vi "Is Enabled.vi"(10 "Plugin in":refnum<class "Plugin.lvclass">) -> (1 "Enabled":bool, 2 "Plugin out":refnum<class "Plugin.lvclass">)   [LabVIEW 2015, in "Plugin.lvclass"]
uses:
  Plugin.lvclass
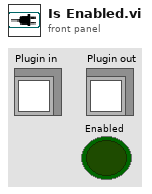
[diagram p1: front panel]
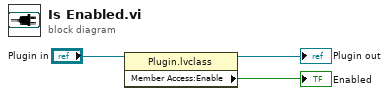
[diagram p0: block diagram]
diagram:
  n1 = property class="Plugin.lvclass"(reference="Plugin in") -> (reference out=→"Plugin out":refnum<class "Plugin.lvclass">, "Member Access:Enable"=→"Enabled":bool)  [unwired: 1 in, 1 out]
